vi "RefreshRankingList.vi"(2 "Arr引用句柄":refnum<vi>, 3 "路径":path) -> ()   [LabVIEW 2019]
uses:
  ctl/InfoOfPlayer.ctl
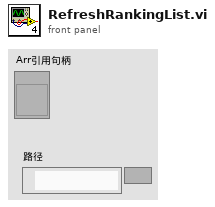
[diagram p1: front panel]
types:
  T1 = typedef "InfoOfPlayer.ctl" = cluster{"得分":i32, "英雄":string}
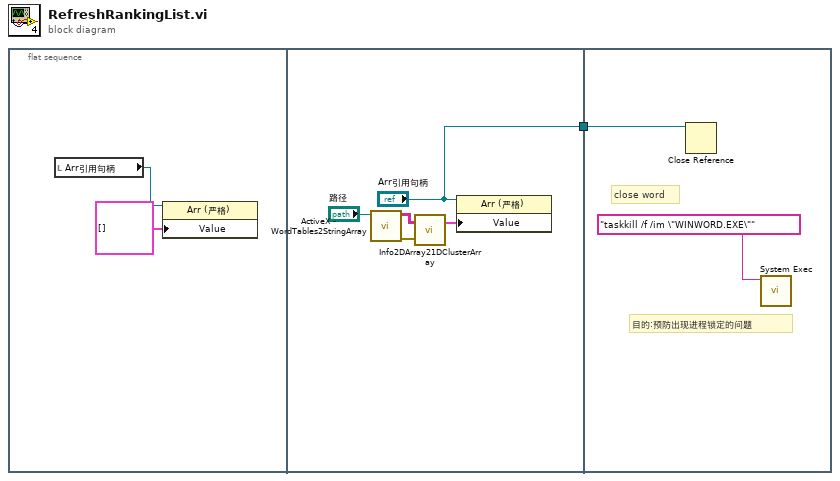
[diagram p0: block diagram]
diagram:
  n1 = flat-sequence {
    tunnel: ["Arr引用句柄"] -> w1
    tunnel: w1 -> [w9]
    frame #0 {
      n2 = local read "Arr引用句柄"() -> (w3:refnum<vi>)
      n3 = property class="Arr (严格)"(reference=w3, "Value"=T1[] [] ("值")) -> ()  [unwired: 1 in, 2 out]
    }
    frame #1 {
      n4 = call "ActiveX - WordTables2StringArray.vi"("File Path Control"="路径") -> ("Error Out"=w8:errorcluster, "Array"=w5:string[][])  [unwired: 7 in, 2 out]
      n5 = call "Info2DArray21DClusterArray.vi"("error in (no error)"=w8, "2DStringArray"=w5) -> ("1DClusterArray"=w6:T1[])  [unwired: 1 out]
      n6 = property class="Arr (严格)"(reference="Arr引用句柄", "Value"=w6) -> ()  [unwired: 1 in, 2 out]
    }
    frame #2 {
      # "目的:预防出现进程锁定的问题"
      # "close word"
      n7 = Close Reference(reference=w9) -> ()  [unwired: 1 in, 1 out]
      n8 = call <vilib>:"System Exec.vi"("command line"="taskkill /f /im \"WINWORD.EXE\"") -> ()  [unwired: 7 in, 4 out]
    }
  }
